vi "Get_frequency_from_waveform.vi"(11 "Waveform Data":waveform(dbl)) -> (2 "Phase":dbl, 3 "Frequency":dbl)   [LabVIEW 2015]
uses:
  <vilib>/express/express analysis/Spectral/Block/exnSpectralBlock spectral measurements RMS poly.vi
  <vilib>/express/express analysis/Spectral/Block/exnSpectralBlock spectral measurements RMS WFM.vi
  <vilib>/express/express analysis/Spectral/XNode/ExpressSpectralMeasurementsBlockNode.xnode
  <vilib>/Analysis/NI_AALPro.lvlib
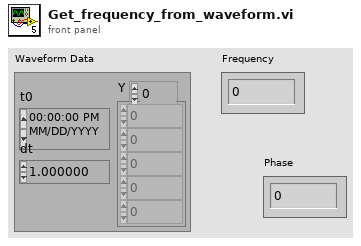
[diagram p1: front panel]
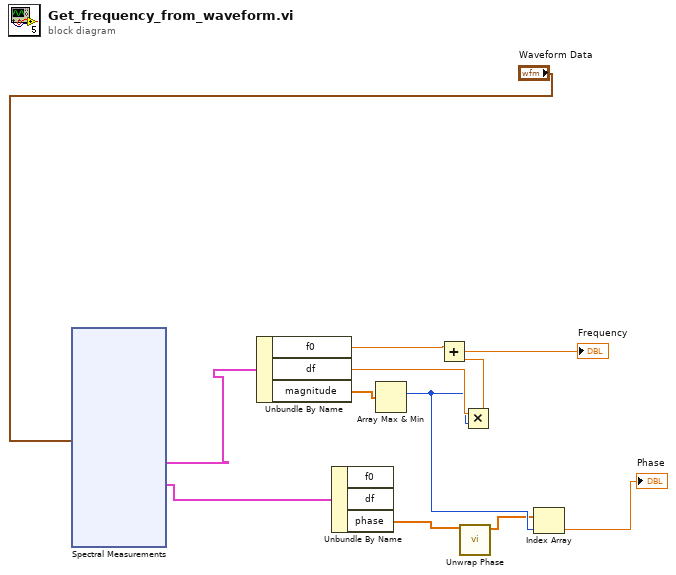
[diagram p0: block diagram]
diagram:
  n1 = xnode "Spectral Measurements"("Signals"="Waveform Data") -> ("FFT - (RMS)"=w6:cluster{"f0":dbl, "df":dbl, "magnitude":dbl[]}, "Phase"=w5:cluster{"f0":dbl, "df":dbl, "phase":dbl[]})  [unwired: 1 in, 1 out]
  n2 = Unbundle By Name(w6) -> ("f0"=w8:dbl, "df"=w9:dbl, "magnitude"=w7:dbl[])
  n3 = Unbundle By Name(w5) -> ("phase"=w1:dbl[])  [unwired: 2 out]
  n4 = Array Max & Min(array=w7) -> (max index (indices)=w4:i32)  [unwired: 3 out]
  n5 = call <vilib>:"Unwrap Phase.vi"("Phase"=w1) -> ("Unwrapped Phase"=w2:dbl[])  [unwired: 9 in, 1 out]
  n6 = Multiply(x=w9, y=w4) -> (x*y=w10:dbl)
  n7 = Add(x=w8, y=w10) -> (x+y=→"Frequency":dbl)
  n8 = Index Array(array=w2, index=w4) -> (element=→"Phase":dbl)
